vi "KB-RS232-MessageDealWithFor Laser.vi"(11 "Receive Message":string="%01$RCS0000100023000010000011\n") -> (0 "TestStartSignal":bool, 1 "Step Number":string, 2 "Motion Done":bool, 3 "EMG":bool)   [LabVIEW 2015]
panel:
  out "已删除元素的数组子集 2":string[](array[string])
  out "反转的数组":string[](array[string])
  out "长度":i32
  out "数组 4":i32[](array[numeric])
  out "数组 3":string[](array[string])
  out "数组 2":string[][](array[string])
  out "x/y":dbl
  out "大小":i32
  out "已删除元素的数组子集":string[](array[string])
  out "数组":string[](array[string])
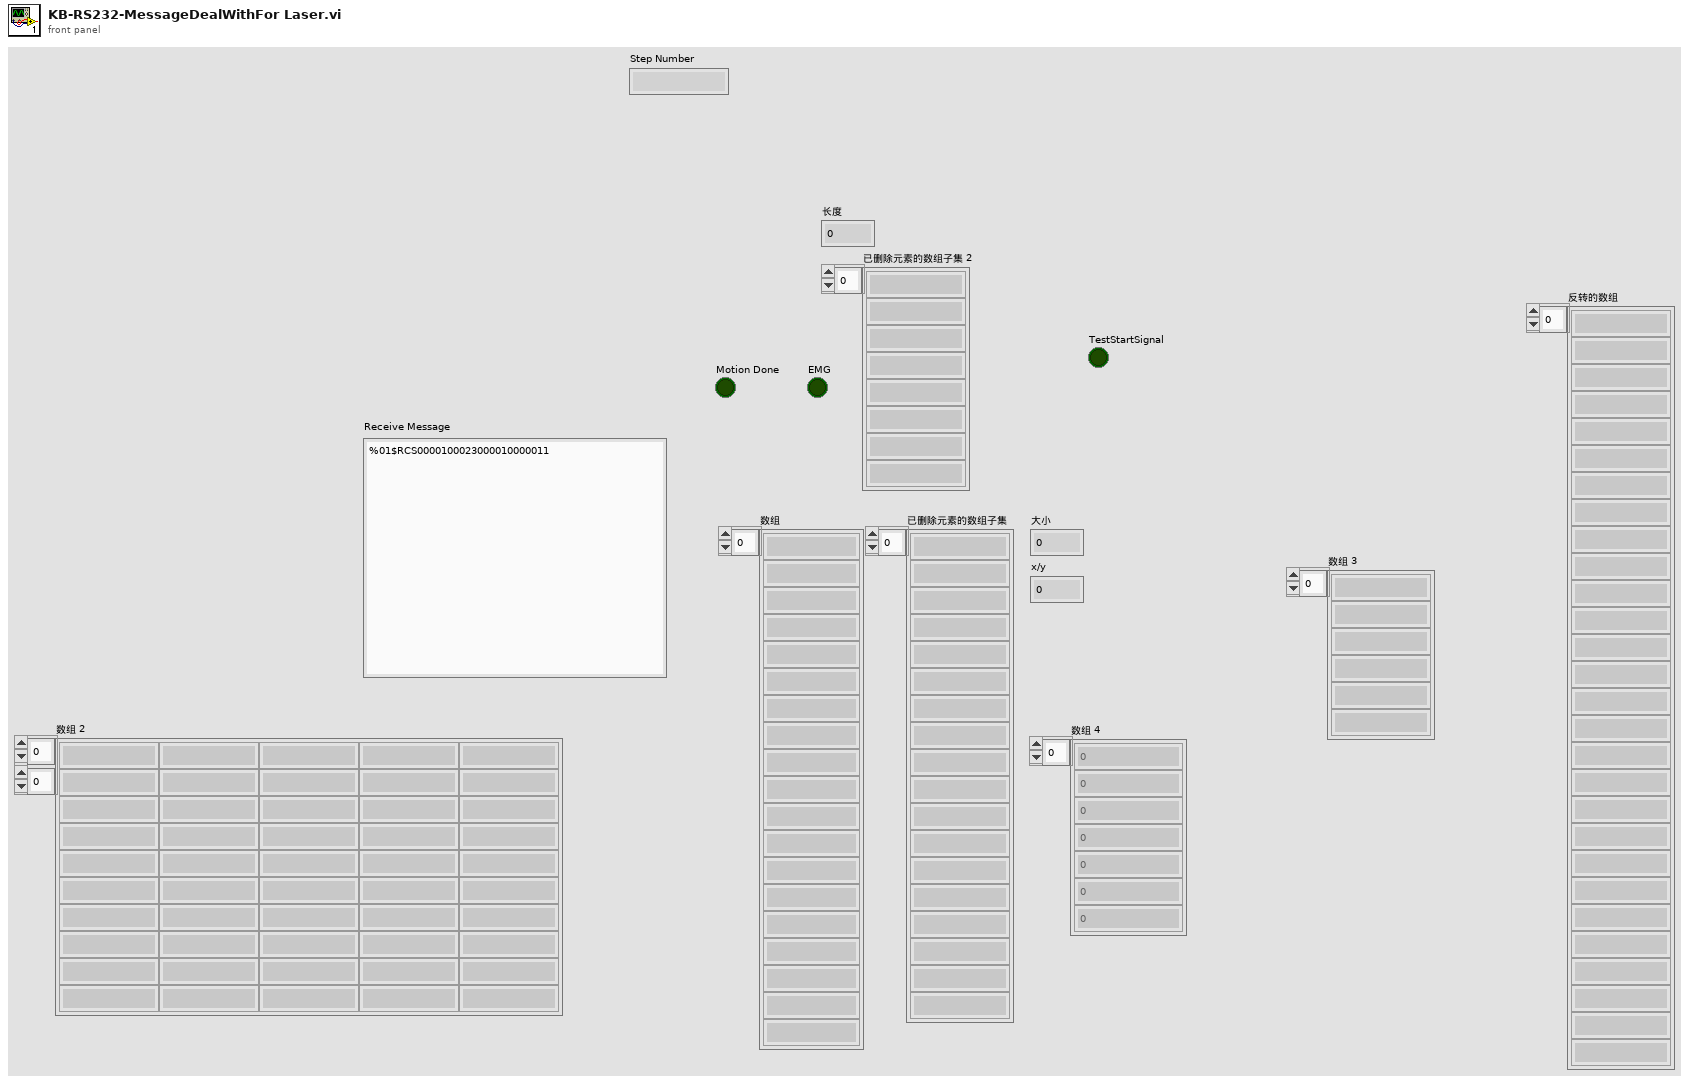
[diagram p1: front panel]
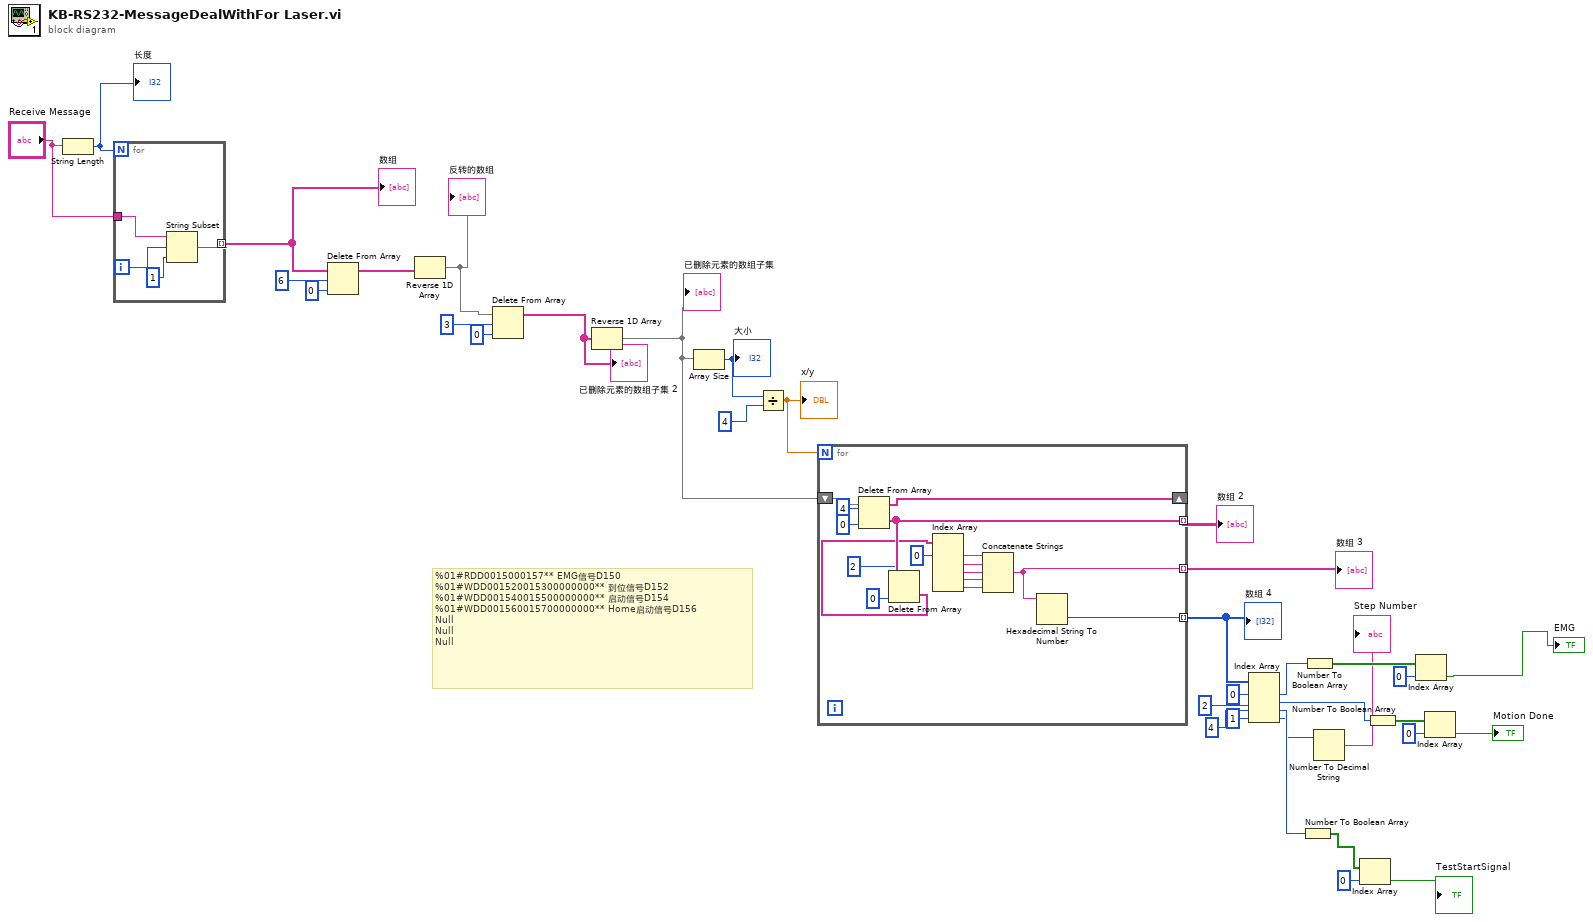
[diagram p0: block diagram]
diagram:
  # "%01#RDD0015000157**\tEMG信号D150\n%01#WDD001520015300000000**\t到位信号D152\n%01#WDD001540015500000000**\t启动信号D154\n%01#WDD001560015700000000**\tHome启动信号D156\nNull\t\nNull\t\nNull"
  n1 = String Length(string="Receive Message") -> (length=w35:i32)
  "长度" <- w35
  n2 = for {
    N: w35 -> [_]
    tunnel: "Receive Message" -> [w39]
    tunnel: [w36] -> w33 mode=indexing
    i -> [w38]
    n3 = String Subset(string=w39, offset (0)=w38, length (rest)=1 ("长度（剩余）")) -> (substring=w36:string)
  }
  "数组" <- w33
  n4 = Delete From Array(array=w33, length=6 ("长度"), index=0 ("索引")) -> (array with subset deleted=w30:string[])  [unwired: 1 out]
  n5 = Reverse 1D Array(array=w30) -> (reversed array=w27:string[])
  "反转的数组" <- w27
  n6 = Delete From Array(array=w27, length=3 ("长度"), index=0 ("索引")) -> (array with subset deleted=w26:string[])  [unwired: 1 out]
  "已删除元素的数组子集 2" <- w26
  n7 = Reverse 1D Array(array=w26) -> (reversed array=w22:string[])
  "已删除元素的数组子集" <- w22
  n8 = Array Size(array=w22) -> (size(s)=w25:i32)
  "大小" <- w25
  n9 = Divide(x=w25, y=4) -> (x/y=w23:dbl)
  "x/y" <- w23
  n10 = for {
    N: w23 -> [_]
    shift-right: [w52] -> _
    shift-left: w22 -> [w55]
    tunnel: [w43] -> w21 mode=indexing
    tunnel: [w46] -> w20 mode=indexing
    tunnel: [w45] -> w19 mode=indexing
    n11 = Delete From Array(array=w55, length=4 ("长度"), index=0 ("索引")) -> (deleted portion=w43:string[], array with subset deleted=w52:string[])
    n12 = Delete From Array(array=w43, length=2 ("长度"), index=0 ("索引")) -> (deleted portion=w40:string[])  [unwired: 1 out]
    n13 = Index Array(array=w40, index #1=0 ("索引")) -> (element #1=w50:string, element #2=w49:string, element #3=w48:string, element #4=w47:string, element #5=w44:string)  [unwired: 4 in]
    n14 = Concatenate Strings(w50, w49, w48, w47, w44) -> (w46:string)
    n15 = Hexadecimal String To Number(string=w46) -> (number=w45:u32)  [unwired: 2 in, 1 out]
  }
  "数组 2" <- w21
  "数组 3" <- w20
  "数组 4" <- w19
  n16 = Index Array(array=w19, index #1=0 ("索引"), index #2=2 ("索引"), index #3=4 ("索引"), index #4=1 ("索引")) -> (element #1=w17:u32, element #2=w7:u32, element #3=w5:u32, element #4=w3:u32)
  n17 = Number To Boolean Array(number=w5) -> (Boolean array=w11:bool[])
  n18 = Number To Boolean Array(number=w17) -> (Boolean array=w16:bool[])
  n19 = Number To Decimal String(number=w3) -> (decimal integer string=→"Step Number":string)  [unwired: 1 in]
  n20 = Index Array(array=w11, index=0 ("索引")) -> (element=→"TestStartSignal":bool)
  n21 = Number To Boolean Array(number=w7) -> (Boolean array=w13:bool[])
  n22 = Index Array(array=w16, index=0 ("索引")) -> (element=→"EMG":bool)
  n23 = Index Array(array=w13, index=0 ("索引")) -> (element=→"Motion Done":bool)
